vi "GenerateReceipt.vi"(8 "error in (no error)":errorcluster, 11 "STOMP in":refnum<class "STOMP.lvclass">) -> (0 "error out":errorcluster, 2 "Receipt Header":T1, 3 "STOMP out":refnum<class "STOMP.lvclass">)   [LabVIEW 2017, in "LabVIEW STOMP.lvlib" / "STOMP.lvclass"]
uses:
  STOMP.lvclass
  Typedefs/Type_FrameHeader.ctl
  STOMP.lvclass/STOMP.ctl
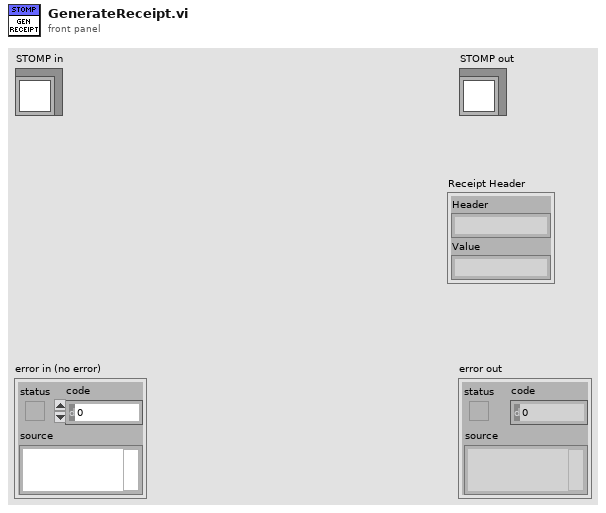
[diagram p1: front panel]
types:
  T1 = typedef "LabVIEW STOMP.lvlib/STOMP.lvclass/Type_FrameHeader.ctl" = cluster{"Header":string, "Value":string}
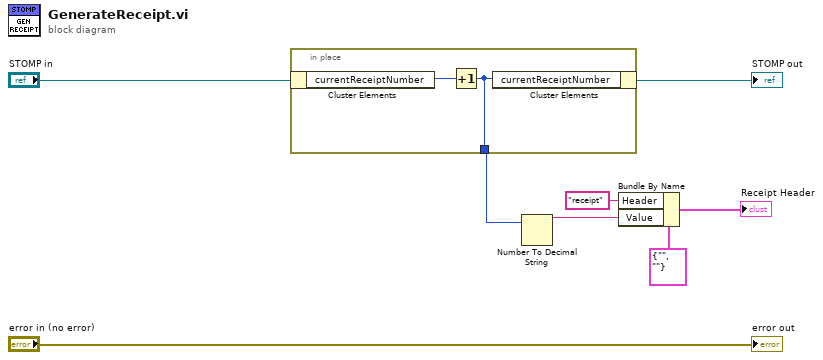
[diagram p0: block diagram]
diagram:
  n1 = in-place {
    in-place-border: [w9] -> w2
    n2 = in-place-cluster #1("STOMP in") -> ("currentReceiptNumber"=w10:u64)
    n3 = Increment(x=w10) -> (x+1=w9:u64)
    n4 = in-place-cluster #1("currentReceiptNumber"=w9) -> (→"STOMP out":refnum<class "STOMP.lvclass">)
  }
  n5 = Number To Decimal String(number=w2) -> (decimal integer string=w1:string)  [unwired: 1 in]
  n6 = Bundle By Name(cluster=T1 {"Header"="", "Value"=""} ("Type_FrameHeader"), "Header"="receipt", "Value"=w1) -> (→"Receipt Header":T1)
  "error out" <- "error in (no error)"
